vi "Consume Memory.vi"() -> ()   [LabVIEW 2016]
panel:
  in  "stop":bool
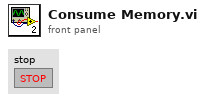
[diagram p1: front panel]
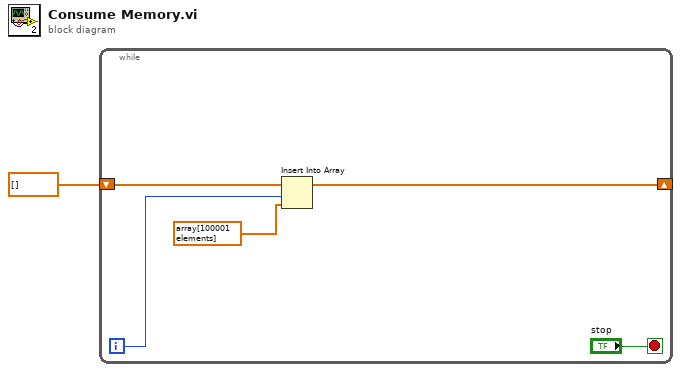
[diagram p0: block diagram]
diagram:
  n1 = while {
    shift-right: [w4] -> _
    shift-left: dbl[] [] -> [w5]
    i -> [w2]
    stop <- "stop" stop-if-true
    n2 = Insert Into Array(array=w5, index=w2, new element=dbl[] array[100001 elements]) -> (w4:dbl[])
  }
